vi "Path Notation End Name.vi"(11 "Item Path":string) -> (1 "Number of Paths":i32, 2 "<JSON>End Name":string)   [LabVIEW 2017, in "JSONtext.lvlib"]
uses:
  JSONtext.lvlib
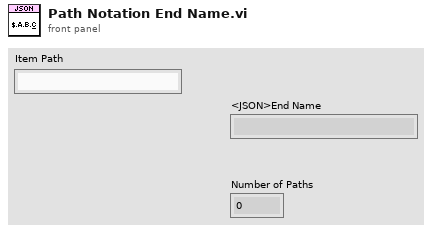
[diagram p1: front panel]
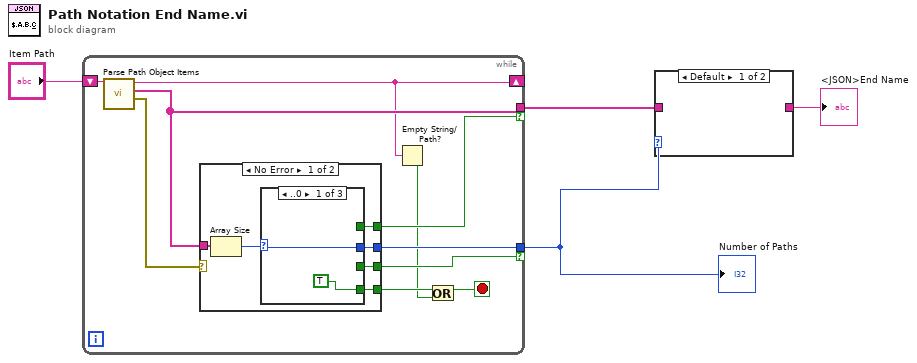
[diagram p0: block diagram]
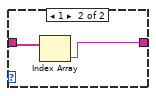
[diagram p2: hidden frame]
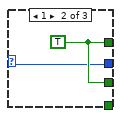
[diagram p3: hidden frame]
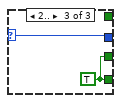
[diagram p4: hidden frame]
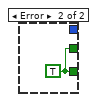
[diagram p5: hidden frame]
diagram:
  n1 = while {
    shift-right: [w7] -> _
    shift-left: "Item Path" -> [w14]
    tunnel: [w13] -> w2 if=w12
    tunnel: [w10] -> w1 if=w9
    stop <- w6 stop-if-true
    n2 = call "Parse Path Object Items.vi"("Path with leading Object element"=w14) -> ("error out"=w8:errorcluster, "<JSON>items names"=w13:string[], "Rest or Path"=w7:string)  [unwired: 8 in]
    n3 = case shown="No Error" w8 {
      tunnel: w13 -> [w20 _]
      tunnel: [w18 _] -> w12
      tunnel: [w17 w27] -> w11
      tunnel: [w16 _] -> w10
      tunnel: [w15 w27] -> w9
      frame No Error {
        n4 = Array Size(array=w20) -> (size(s)=w19:i32)
        n5 = case shown="..0" w19 {
          selector: w19 -> [w21 w23 w25]
          tunnel: [_ w24 _] -> w18
          tunnel: [TRUE _ w26] -> w17
          tunnel: [w21 w23 w25] -> w16
          tunnel: [_ w24 w26] -> w15
          frame ..0 {
          }
          frame 1 {
            w24 = TRUE
          }
          frame 2.. {
            w26 = TRUE
          }
        }
      }
      frame Error {
        w27 = TRUE
      }
    }
    n6 = Empty String/Path?(string/path=w7) -> (empty?=w5:bool)
    n7 = Or(x=w11, y=w5) -> (x .or. y?=w6:bool)
  }
  "Number of Paths" <- w1
  n8 = case shown="Default" w1 {
    tunnel: w2 -> [_ w29]
    tunnel: [_ w28] -> w3
    frame Default {
    }
    frame 1 {
      n9 = Index Array(array=w29) -> (element=w28:string)  [unwired: 1 in]
    }
  }
  "<JSON>End Name" <- w3
